vi "C4Buf_getDataPartFloat.vi"(0 "c4buf in":refnum<k24>, 5 "partIdx in":i64, 11 "error in (no error)":errorcluster) -> (4 "c4buf out":refnum<k24>, 6 "data out":dbl[][](array[numeric]), 15 "error out":errorcluster)   [LabVIEW 2015, in "libC4HdlLV.lvlib"]
uses:
  libC4HdlLV.lvlib
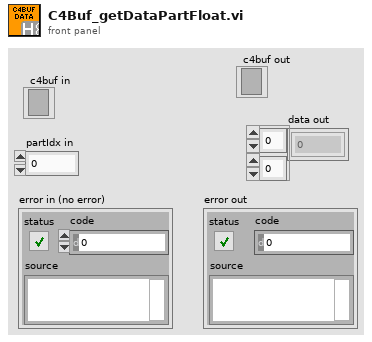
[diagram p1: front panel]
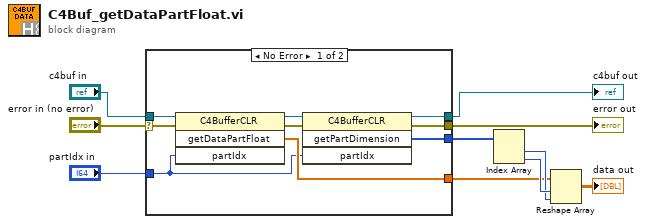
[diagram p0: block diagram]
diagram:
  n1 = case shown="No Error" "error in (no error)" {
    selector: "error in (no error)" -> [w12 w21]
    tunnel: [w19 _] -> w8
    tunnel: [w18 _] -> w7
    tunnel: "partIdx in" -> [w17 _]
    tunnel: "c4buf in" -> [w11 w20]
    tunnel: [w14 w21] -> w5
    tunnel: [w13 w20] -> w2
    frame No Error {
      n2 = invoke class="C4BufferCLR" method="getDataPartFloat"(reference=w11, error in=w12, "partIdx"=w17) -> (reference out=w16:refnum<k24>, error out=w15:errorcluster, "getDataPartFloat"=w19:dbl[])  [unwired: 1 in, 1 out]
      n3 = invoke class="C4BufferCLR" method="getPartDimension"(reference=w16, error in=w15, "partIdx"=w17) -> (reference out=w13:refnum<k24>, error out=w14:errorcluster, "getPartDimension"=w18:i64[])  [unwired: 1 in, 1 out]
    }
    frame Error {
    }
  }
  "error out" <- w5
  "c4buf out" <- w2
  n4 = Index Array(array=w7) -> (element #1=w9:i64, element #2=w10:i64)  [unwired: 2 in]
  n5 = Reshape Array(w8, w10, w9) -> (→"data out":dbl[][])
